vi "clone.vi"(0 "reference":refnum<class "StateTransitionEdge.lvclass">, 5 "error in (no error)":errorcluster) -> (14 "reference out":refnum<class "StateTransitionEdge.lvclass">, 15 "clonedEdge":refnum<class "AbstractEdge.lvclass">, 19 "error out":errorcluster)   [LabVIEW 2020, in "StateTransitionEdge.lvclass"]
doc: "clone"
uses:
  <resource>/Framework/Providers/Open_GDS/UML/StateTransitionEdge_class/StateTransitionEdge.lvclass
  C:/Program Files (x86)/National Instruments/LabVIEW 2020/resource/Framework/Providers/Open_GDS/UML/ClassRelationshipEdge_class/ClassRelationshipEdge.lvclass
  C:/Program Files (x86)/National Instruments/LabVIEW 2020/resource/Framework/Providers/Open_GDS/UML/SegmentedLineEdge_class/SegmentedLineEdge.lvclass
  C:/Program Files (x86)/National Instruments/LabVIEW 2020/resource/Framework/Providers/Open_GDS/UML/GeneralPathEdge_class/GeneralPathEdge.lvclass
  C:/Program Files (x86)/National Instruments/LabVIEW 2020/resource/Framework/Providers/Open_GDS/UML/AbstractEdge_class/AbstractEdge.lvclass
  <resource>/Framework/Providers/Open_GDS/UML/AbstractEdge_class/AbstractEdge.lvclass
  <resource>/Framework/Providers/Open_GDS/UML/ClassRelationshipEdge_class/ClassRelationshipEdge.lvclass
  <resource>/Framework/Providers/Open_GDS/UML/SegmentedLineEdge_class/SegmentedLineEdge.lvclass
  <resource>/Framework/Providers/Open_GDS/UML/GeneralPathEdge_class/GeneralPathEdge.lvclass
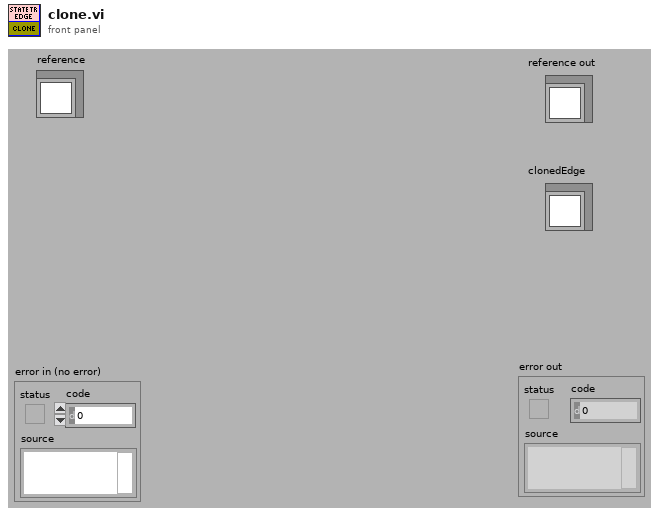
[diagram p1: front panel]
types:
  T1 = typedef "StateTransitionEdge.lvclass/ObjectAttributes.ctl" = cluster{"angle":dbl}
  T2 = typedef "ClassRelationshipEdge.lvclass/ObjectAttributes.ctl" = cluster{"bentStyleRef":refnum<class "BentStyle.lvclass">, "startConnectionOffset":cluster{"x":i32, "y":i32}, "endConnectionOffset":cluster{"x":i32, "y":i32}, "MidLineOffset":cluster{"x":i32, "y":i32}, "DepClass":T3}
  T3 = typedef "ReversedEngineering_ViDependencyDetailsType.ctl" = cluster{"ThisVIs/Ctls":path[], "Dependent_VIs/Ctls":path[]}
  T4 = typedef "SegmentedLineEdge.lvclass/ObjectAttributes.ctl" = cluster{"lineStyle":refnum<class "LineStyle.lvclass">, "startArrowHead":refnum<class "ArrowHead.lvclass">, "endArrowHead":refnum<class "ArrowHead.lvclass">, "startLabel":string, "midLabel":string, "endLabel":string, "MidLabelOffset":T5, "SplitWire":bool}
  T5 = typedef "Point Point2D.ctl" = cluster{"x":dbl, "y":dbl}
  T6 = typedef "GeneralPathEdge.lvclass/ObjectAttributes.ctl" = cluster{"None":bool}
  T7 = typedef "AbstractEdge.lvclass/ObjectAttributes.ctl" = cluster{"start":refnum<class "AbstractNode.lvclass">, "end":refnum<class "AbstractNode.lvclass">}
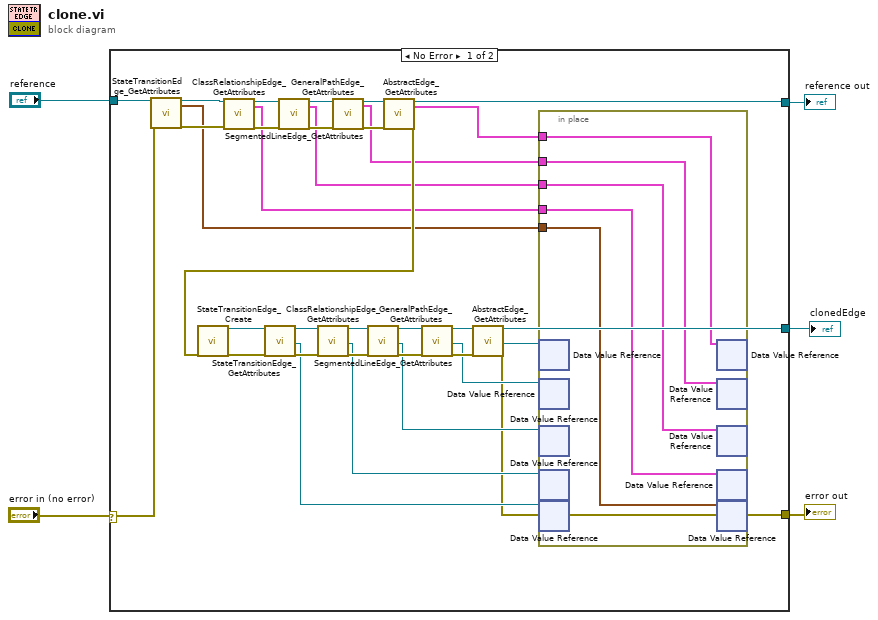
[diagram p0: block diagram]
diagram:
  n1 = case shown="No Error" "error in (no error)" {
    selector: "error in (no error)" -> [w37 w45]
    tunnel: "reference" -> [w39 w46]
    tunnel: [w6 w45] -> w4
    tunnel: [w8 w46] -> w3
    tunnel: [w7 _] -> w1
    frame No Error {
      n2 = call <resource>:"StateTransitionEdge_GetAttributes.vi"("reference in"=w39, "error in (no error)"=w37) -> ("reference out"=w35:refnum<class "StateTransitionEdge.lvclass">, "Data"=w18:T1, "error out"=w34:errorcluster)  [unwired: 1 in, 14 out]
      n3 = call <resource>:"ClassRelationshipEdge_GetAttributes.vi"("reference in"=w35, "error in (no error)"=w34) -> ("reference out"=w31:refnum<class "StateTransitionEdge.lvclass">, "Data"=w17:T2, "error out"=w30:errorcluster)  [unwired: 1 in, 14 out]
      n4 = call <resource>:"SegmentedLineEdge_GetAttributes.vi"("reference in"=w31, "error in (no error)"=w30) -> ("reference out"=w27:refnum<class "StateTransitionEdge.lvclass">, "Data"=w16:T4, "error out"=w26:errorcluster)  [unwired: 1 in, 14 out]
      n5 = call <resource>:"GeneralPathEdge_GetAttributes.vi"("reference in"=w27, "error in (no error)"=w26) -> ("reference out"=w29:refnum<class "StateTransitionEdge.lvclass">, "Data"=w15:T6, "error out"=w28:errorcluster)  [unwired: 14 in, 1 out]
      n6 = call <resource>:"AbstractEdge_GetAttributes.vi"("reference in"=w29, "error in (no error)"=w28) -> ("reference out"=w8:refnum<class "StateTransitionEdge.lvclass">, "Data"=w14:T7, "error out"=w25:errorcluster)  [unwired: 14 in, 1 out]
      n7 = call <resource>:"StateTransitionEdge_Create.vi"("error in (no error)"=w25) -> ("reference out"=w36:refnum<class "StateTransitionEdge.lvclass">, "error out"=w38:errorcluster)  [unwired: 17 in]
      n8 = call <resource>:"StateTransitionEdge_GetAttributes.vi"("reference in"=w36, "error in (no error)"=w38) -> ("reference out"=w33:refnum<class "StateTransitionEdge.lvclass">, "DataRef"=w10:refnum<data-value>, "error out"=w32:errorcluster)  [unwired: 14 in, 1 out]
      n9 = call <resource>:"ClassRelationshipEdge_GetAttributes.vi"("reference in"=w33, "error in (no error)"=w32) -> ("reference out"=w20:refnum<class "StateTransitionEdge.lvclass">, "DataRef"=w11:refnum<data-value>, "error out"=w19:errorcluster)  [unwired: 1 in, 14 out]
      n10 = call <resource>:"SegmentedLineEdge_GetAttributes.vi"("reference in"=w20, "error in (no error)"=w19) -> ("reference out"=w23:refnum<class "StateTransitionEdge.lvclass">, "DataRef"=w12:refnum<data-value>, "error out"=w24:errorcluster)  [unwired: 1 in, 14 out]
      n11 = call <resource>:"GeneralPathEdge_GetAttributes.vi"("reference in"=w23, "error in (no error)"=w24) -> ("reference out"=w21:refnum<class "StateTransitionEdge.lvclass">, "DataRef"=w9:refnum<data-value>, "error out"=w22:errorcluster)  [unwired: 14 in, 1 out]
      n12 = call <resource>:"AbstractEdge_GetAttributes.vi"("reference in"=w21, "error in (no error)"=w22) -> ("reference out"=w7:refnum<class "StateTransitionEdge.lvclass">, "DataRef"=w13:refnum<data-value>, "error out"=w6:errorcluster)  [unwired: 14 in, 1 out]
      n13 = in-place {
        in-place-border: w17 -> [w44]
        in-place-border: w16 -> [w43]
        in-place-border: w15 -> [w42]
        in-place-border: w18 -> [w41]
        in-place-border: w14 -> [w40]
        n14 = in-place-dvr #1(w13) -> ()  [unwired: 2 out]
        n15 = in-place-dvr #2(w9) -> ()  [unwired: 2 out]
        n16 = in-place-dvr #3(w12) -> ()  [unwired: 2 out]
        n17 = in-place-dvr #4(w11) -> ()  [unwired: 2 out]
        n18 = in-place-dvr #5(w10) -> ()  [unwired: 2 out]
        n19 = in-place-dvr #1(w40) -> ()  [unwired: 2 out]
        n20 = in-place-dvr #2(w42) -> ()  [unwired: 2 out]
        n21 = in-place-dvr #3(w43) -> ()  [unwired: 2 out]
        n22 = in-place-dvr #4(w44) -> ()  [unwired: 2 out]
        n23 = in-place-dvr #5(w41) -> ()  [unwired: 2 out]
      }
    }
    frame Error {
    }
  }
  "reference out" <- w3
  "error out" <- w4
  "clonedEdge" <- w1
